vi "VCS Set Homing Parameter.vi"(8 "error in (no error)":errorcluster, 10 "homingParameter":T1, 11 "axis in":cluster{"keyHandle":u32, "nodeId":u16}={"keyHandle"=0, "nodeId"=1}) -> (0 "error out":errorcluster, 3 "axis out":cluster{"keyHandle":u32, "nodeId":u16}={"keyHandle"=0, "nodeId"=1})   [LabVIEW 2019, in "maxonEPOS.lvlib"]
doc: "<B>VCS Set Homing Parameter</B> writes all homing parameters."
uses:
  Examples/maxonEPOS.lvlib
  Resources/EposCmd.dll
  Resources/EposCmd64.dll
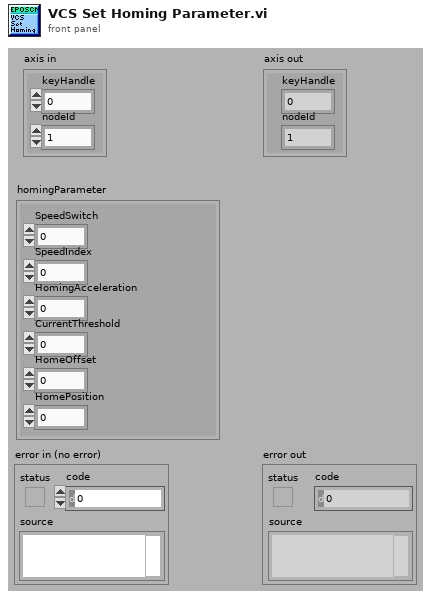
[diagram p1: front panel]
types:
  T1 = cluster{"SpeedSwitch":u32, "SpeedIndex":u32, "HomingAcceleration":u32, "CurrentThreshold":u16, "HomeOffset":i32, "HomePosition":i32}
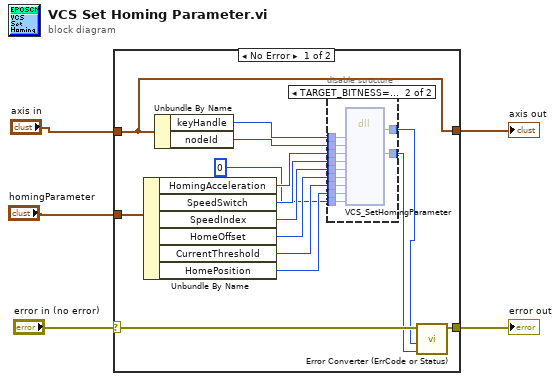
[diagram p0: block diagram]
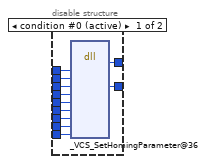
[diagram p2: hidden frame]
diagram:
  n1 = case shown="No Error" "error in (no error)" {
    selector: "error in (no error)" -> [w20 w44]
    tunnel: [w19 w44] -> w4
    tunnel: "axis in" -> [w8 w43]
    tunnel: "homingParameter" -> [w15 _]
    tunnel: [w8 w43] -> w1
    frame No Error {
      n2 = Unbundle By Name(w15) -> ("HomingAcceleration"=w14:u32, "SpeedSwitch"=w13:u32, "SpeedIndex"=w12:u32, "HomeOffset"=w11:i32, "CurrentThreshold"=w10:u16, "HomePosition"=w9:i32)
      n3 = Unbundle By Name(w8) -> ("keyHandle"=w17:u32, "nodeId"=w16:u16)
      n4 = disable-structure shown="TARGET_BITNESS==64" {
        disable-tunnel: [w31 w42] -> w18
        disable-tunnel: w17 -> [w30 w41]
        disable-tunnel: w16 -> [w29 w40]
        disable-tunnel: w14 -> [w28 w39]
        disable-tunnel: w13 -> [w27 w38]
        disable-tunnel: w12 -> [w26 w37]
        disable-tunnel: w11 -> [w25 w36]
        disable-tunnel: w10 -> [w24 w35]
        disable-tunnel: w9 -> [w23 w34]
        disable-tunnel: u32 0 ("pErrorCode") -> [w22 w33]
        disable-tunnel: [w21 w32] -> w6
        frame condition #0 (active) {
          n5 = dll-call lib="C:/workspace/project/scancon/sw/SSI_Tool/InstrumentsInterfaces/Motordriver/maxon EPOS/Resources/EposCmd.*" fn="_VCS_SetHomingParameter@36"("KeyHandle"=w30, "NodeId"=w29, "HomingAcceleration"=w28, "SpeedSwitch"=w27, "SpeedIndex"=w26, "HomeOffset"=w25, "CurrentThreshold"=w24, "HomePosition"=w23, "pErrorCode"=w22) -> (w21:i32, "pErrorCode"=w31:u32)  [unwired: 11 in, 2 out]
        }
        frame condition #1 {
          n6 = dll-call lib="C:/Sources/LabView/maxon EPOS/Resources/EposCmd64.*" fn="VCS_SetHomingParameter" ("EposCmd.dll:_VCS_SetHomingParameter@36")("KeyHandle"=w41, "NodeId"=w40, "HomingAcceleration"=w39, "SpeedSwitch"=w38, "SpeedIndex"=w37, "HomeOffset"=w36, "CurrentThreshold"=w35, "HomePosition"=w34, "pErrorCode"=w33) -> ("Rückgabetyp"=w32:i32, "pErrorCode"=w42:u32)  [unwired: 11 in, 2 out]
        }
      }
      n7 = call "Error Converter (ErrCode or Status).vi"("error code"=w18, "return type"=w6, "error in (no error)"=w20) -> ("error out"=w19:errorcluster)  [unwired: 7 in]
    }
    frame Error {
    }
  }
  "error out" <- w4
  "axis out" <- w1
